vi "Update Calibration.vi"   [LabVIEW 2017, in "nisyscfg.lvlib"]
doc: "Updates the external calibration information for a device. You can only use this VI to update calibration information if the Supports Calibration Write property is TRUE."
uses:
  <vilib>/nisyscfg/nisyscfg.lvlib
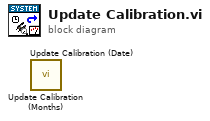
[diagram p0: block diagram]
diagram:
  n1 = call <vilib>:"Update Calibration (Months).vi"() -> ()  [unwired: 9 in, 3 out]
  n2 = call <vilib>:"Update Calibration (Date).vi"() -> ()  [unwired: 9 in, 3 out]
